vi "create new obj.vi"(7 "clock rate":u8(ring) items=["1M", "2M", "3M", "400k"], 8 "error in (no error)":errorcluster caption="에러 입력(에러 없음)", 9 "data byte":u8=1, 10 "address byte":u8=1, 11 "slave address":u8 format="%02x") -> (0 "error out":errorcluster caption="에러 출력", 3 "new I2C obj":refnum<class "I2C.lvclass">)   [LabVIEW 2020, in "I2C.lvclass"]
uses:
  I2C.lvclass
  I2C.lvclass/I2C.ctl
  Accessors/Write slave address.vi
  Accessors/Write clock rate.vi
  Accessors/Write address byte.vi
  Accessors/Write data byte.vi
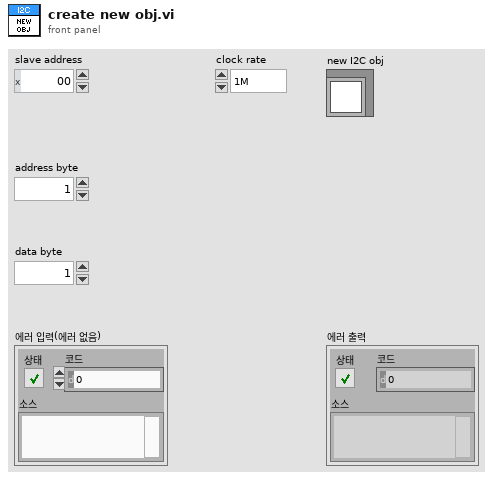
[diagram p1: front panel]
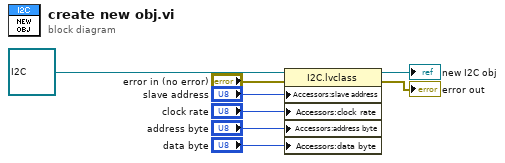
[diagram p0: block diagram]
diagram:
  n1 = property class="I2C.lvclass"(reference=refnum<class "I2C.lvclass"> refnum ("I2C.lvclass"), error in="error in (no error)", "Accessors:slave address"="slave address", "Accessors:clock rate"="clock rate", "Accessors:address byte"="address byte", "Accessors:data byte"="data byte") -> (reference out=→"new I2C obj":refnum<class "I2C.lvclass">, error out=→"error out":errorcluster)
